vi "Newton Raphson Zero Finder (Formula).vi"(7 "accuracy":dbl=1e-08 format="%.2e", 8 "formula":string, 9 "end":dbl=1.0 format="%.2f", 10 "start":dbl format="%.2f", 11 "h":dbl=1e-08 format="%.2e") -> (0 "error":i32, 1 "ticks":u32, 2 "f(zero)":dbl format="%.2f", 3 "zero":dbl format="%.2f")   [LabVIEW 2017, in "NI_Gmath.lvlib"]
doc: "Determines a zero of a 1D function close to two points with the help of the derivative of this 1D function. The two values form a search limit for the unknown zero of the 1D function. You must manually select the polymorphic instance to use."
uses:
  <vilib>/gmath/NI_Gmath.lvlib
panel:
  # "Example:\n\n accuracy: 1E-8 \n h: 1E-8 \n start: 0.0\n end: 1.0\n formula: x^2+sin(x)-1"
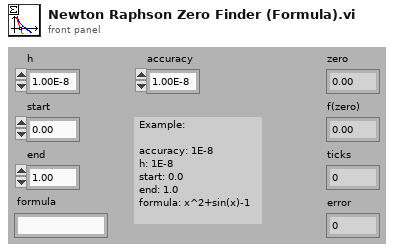
[diagram p1: front panel]
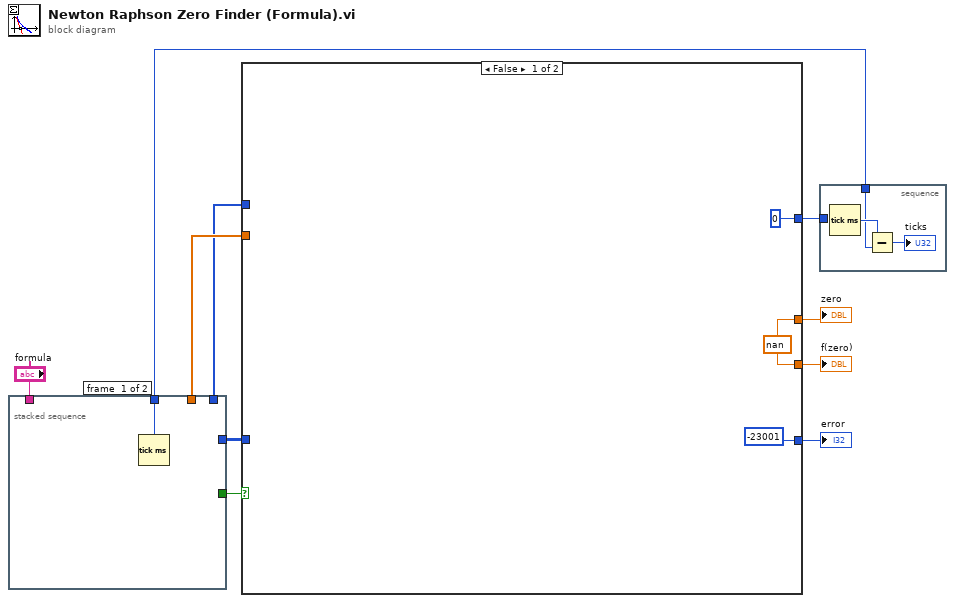
[diagram p0: block diagram]
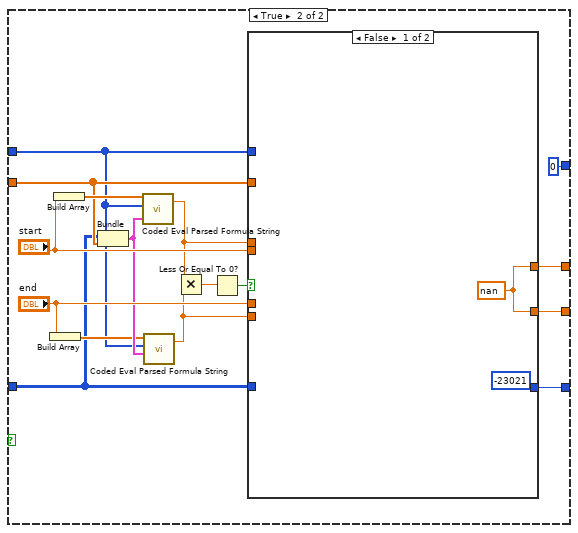
[diagram p2: hidden frame]
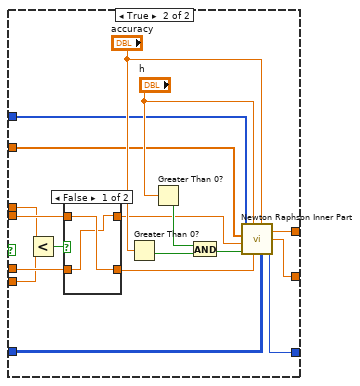
[diagram p3: hidden frame]
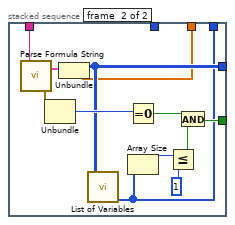
[diagram p5: hidden frame]
diagram:
  n1 = stacked-sequence {
    tunnel: [_ w23] -> w10
    tunnel: [w11 _] -> w8
    tunnel: "formula" -> [_ w16]
    tunnel: [_ w13] -> w3
    tunnel: [_ w12] -> w2
    tunnel: [_ w14] -> w1
    frame #0 {
      n2 = Tick Count (ms)() -> (millisecond timer value=w11:u32)
    }
    frame #1 {
      n3 = call <vilib>:"Parse Formula String.vi"("formula"=w16) -> ("error out"=w18:errorcluster, "Parsed Formula"=w15:cluster{"Table":i32[][], "Y Values":dbl[]})  [unwired: 1 in]
      n4 = Unbundle(w18) -> ("code"=w17:i32)  [unwired: 2 out]
      n5 = Unbundle(w15) -> ("Table"=w14:i32[][], "Y Values"=w13:dbl[])
      n6 = call <vilib>:"List of Variables.vi"("Table"=w14) -> ("List of variables"=w12:i32[])
      n7 = Equal To 0?(x=w17) -> (x = 0?=w22:bool)
      n8 = Array Size(array=w12) -> (size(s)=w19:i32)
      n9 = Less Or Equal?(x=w19, y=1) -> (x <= y?=w21:bool)
      n10 = And(x=w22, y=w21) -> (x .and. y?=w23:bool)
    }
  }
  n11 = case shown="False" w10 {
    tunnel: [0 0] -> w9
    tunnel: [w25 w38] -> w6
    tunnel: [w25 w37] -> w5
    tunnel: [-23001 w36] -> w4
    tunnel: w3 -> [_ w29]
    tunnel: w2 -> [_ w28]
    tunnel: w1 -> [_ w27]
    frame False {
      w25 = nan
    }
    frame True {
      n12 = Build Array("end") -> (w30:dbl[])
      n13 = Build Array("start") -> (w33:dbl[])
      n14 = Bundle("Table"=w27, "Y Values"=w29) -> (w32:cluster{"Table":i32[][], "Y Values":dbl[]})  [unwired: 1 out]
      n15 = call <vilib>:"Coded Eval Parsed Formula String.vi"("Parsed Formula"=w32, "Variables"=w28, "X Values"=w33) -> ("y value"=w35:dbl)  [unwired: 1 in, 1 out]
      n16 = call <vilib>:"Coded Eval Parsed Formula String.vi"("Parsed Formula"=w32, "Variables"=w28, "X Values"=w30) -> ("y value"=w34:dbl)  [unwired: 1 in, 1 out]
      n17 = Multiply(x=w35, y=w34) -> (x*y=w31:dbl)
      n18 = Less Or Equal To 0?(x=w31) -> (x <= 0?=w39:bool)
      n19 = case shown="False" w39 {
        tunnel: "start" -> [_ w51]
        tunnel: "end" -> [_ w50]
        tunnel: [w44 w62] -> w38
        tunnel: [w44 w61] -> w37
        tunnel: [-23021 w55] -> w36
        tunnel: w35 -> [_ w49]
        tunnel: w34 -> [_ w48]
        tunnel: w28 -> [_ w47]
        tunnel: w27 -> [_ w46]
        tunnel: w29 -> [_ w45]
        frame False {
          w44 = nan
        }
        frame True {
          n20 = Less?(x=w49, y=w48) -> (x < y?=w54:bool)
          n21 = case shown="False" w54 {
            tunnel: w51 -> [w64 w66]
            tunnel: w50 -> [w63 w65]
            tunnel: [w63 w66] -> w53
            tunnel: [w64 w65] -> w52
            frame False {
            }
            frame True {
            }
          }
          n22 = Greater Than 0?(x="accuracy") -> (x > 0?=w58:bool)
          n23 = Greater Than 0?(x="h") -> (x > 0?=w57:bool)
          n24 = And(x=w57, y=w58) -> (x .and. y?=w56:bool)
          n25 = call <vilib>:"Newton Raphson Inner Part.vi"("table"=w46, "accuracy"="accuracy", "end/start"=w52, "case"=w56, "start/end"=w53, "h"="h", "result"=w45, "list of variables"=w47) -> ("error"=w55:i32, "zero"=w61:dbl, "f(zero)"=w62:dbl)
        }
      }
    }
  }
  "error" <- w4
  "zero" <- w6
  "f(zero)" <- w5
  n26 = stacked-sequence {
    tunnel: w8 -> [w68]
    tunnel: w9 -> [_]
    frame #0 {
      n27 = Tick Count (ms)() -> (millisecond timer value=w69:u32)
      n28 = Subtract(x=w69, y=w68) -> (x-y=→"ticks":u32)
    }
  }
